vi "GA_Generate_Population.vi"(8 "error in (no error)":errorcluster, 9 "seed":i32=-1, 11 "GA in":refnum<class "GA.lvclass">) -> (0 "error out":errorcluster, 3 "GA out":refnum<class "GA.lvclass">)   [LabVIEW 2013, in "GA.lvclass"]
uses:
  GA.lvclass
  GA.lvclass/GA.ctl
  <vilib>/Analysis/1siggen.llb/Riffle Array (I32).vi
  <vilib>/Analysis/NI_AALBase.lvlib
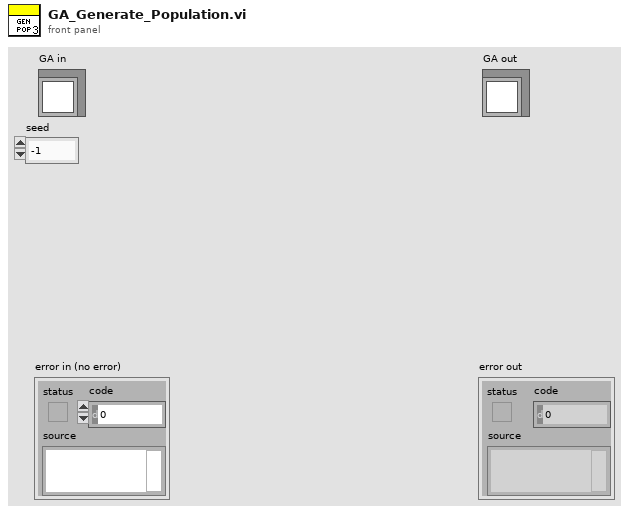
[diagram p1: front panel]
types:
  T1 = typedef "Solution.ctl" = cluster{"Schedule":u16[], "Fitness":u16, "Fitness Valid?":bool}
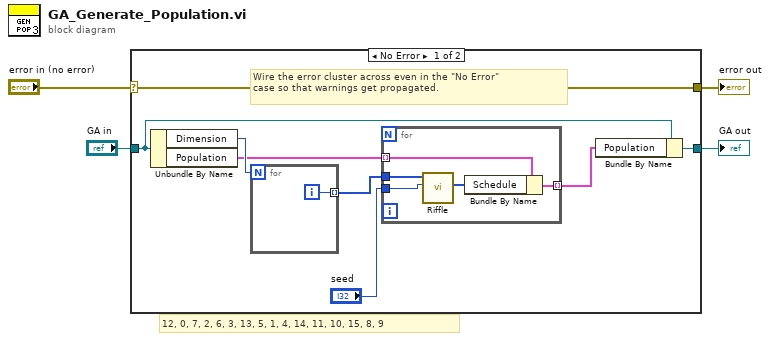
[diagram p0: block diagram]
diagram:
  # "12, 0, 7, 2, 6, 3, 13, 5, 1, 4, 14, 11, 10, 15, 8, 9"
  n1 = case shown="No Error" "error in (no error)" {
    selector: "error in (no error)" -> [w12 w20]
    tunnel: [w12 w20] -> w3
    tunnel: [w8 w19] -> w1
    tunnel: "GA in" -> [w9 w19]
    frame No Error {
      # "Wire the error cluster across even in the \"No Error\"\ncase so that warnings get propagated."
      n2 = Unbundle By Name(w9) -> ("Dimension"=w11:i32, "Population"=w6:T1[])
      n3 = for {
        N: w11 -> [_]
        tunnel: [w13] -> w10 mode=indexing
        i -> [w13]
      }
      n4 = for {
        tunnel: w10 -> [w18]
        tunnel: "seed" -> [w17]
        tunnel: w6 -> [w15] mode=indexing
        tunnel: [w14] -> w5 mode=indexing
        n5 = call-poly <vilib>:"Riffle.vi"("seed"=w17, "X"=w18) -> ("Riffled Index"=w16:i32[])  [unwired: 7 in, 2 out]
        n6 = Bundle By Name(cluster=w15, "Schedule"=w16) -> (w14:T1)
      }
      n7 = Bundle By Name(cluster=w9, "Population"=w5) -> (w8:refnum<class "GA.lvclass">)
    }
    frame Error {
    }
  }
  "error out" <- w3
  "GA out" <- w1
